vi "Teardown.vi"(8 "error in":errorcluster, 11 "_Rescript Msg in":refnum<class "_Msg Rescript.lvclass">) -> (0 "error out":errorcluster)   [LabVIEW 2025, in "_Msg Rescript.lvlib" / "_Msg Rescript.lvclass"]
uses:
  _Msg Rescript.lvclass
  _Msg Rescript.lvclass/_Msg Rescript.ctl
  _Shared/Project Stuff/Project Stuff.lvclass
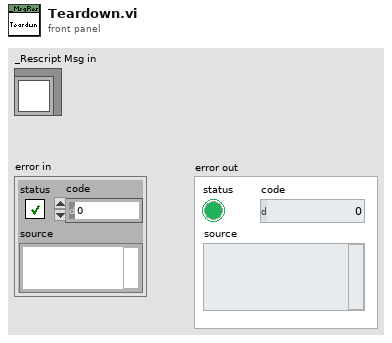
[diagram p1: front panel]
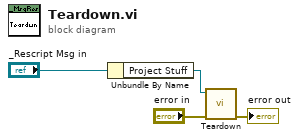
[diagram p0: block diagram]
diagram:
  n1 = Unbundle By Name("_Rescript Msg in") -> ("Project Stuff"=w3:refnum<class "Project Stuff.lvclass">)
  n2 = call "Teardown.vi"("Error in"="error in", "Project Stuff in"=w3) -> ("Error out"=→"error out":errorcluster)  [unwired: 9 in]
